vi "test Scaled Parameters for RT to RT.vi"(8 "error in":errorcluster, 11 "Loopback in":refnum<class "Loopback.lvclass">) -> (0 "error out":errorcluster, 3 "Loopback out":refnum<class "Loopback.lvclass">)   [LabVIEW 2020, in "Loopback.lvclass"]
uses:
  Loopback.lvclass
  <vilib>/NI/VeriStand Custom Device Testing Tools/VeriStandTestUtilities/VeriStandTestUtilities.lvlib
  <vilib>/NI VeriStand/Execution/Workspace/NI_VS Workspace ExecutionAPI.lvlib
  <vilib>/NI VeriStand/Execution/Workspace/NI VeriStand - Set Multiple Channel Values.vi
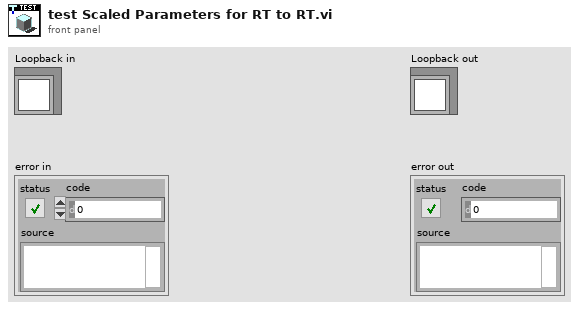
[diagram p1: front panel]
types:
  T1 = typedef "NI_VS Workspace ExecutionAPI.lvlib/WorkspaceAPI.ctl" = refnum<k24>
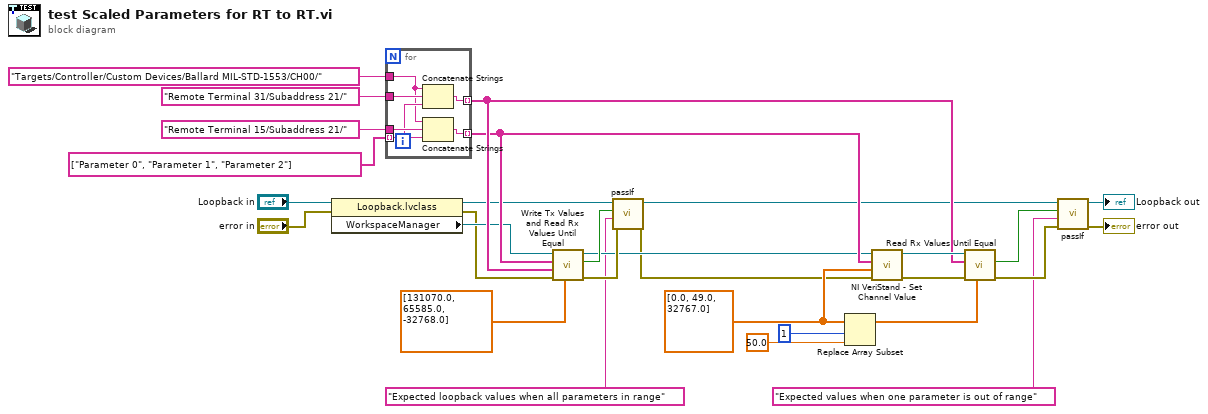
[diagram p0: block diagram]
diagram:
  w27 = dbl[] [0.0, 49.0, 32767.0] ("appended array")
  n1 = property class="Loopback.lvclass"(reference="Loopback in", error in="error in") -> (reference out=w3:refnum<class "Loopback.lvclass">, error out=w4:errorcluster, "WorkspaceManager"=w5:T1)
  n2 = for {
    tunnel: "Remote Terminal 15/Subaddress 21/" ("Channel") -> [w34]
    tunnel: string[] ["Parameter 0", "Parameter 1", "Parameter 2"] ("Channels") -> [w33] mode=indexing
    tunnel: [w35] -> w20 mode=indexing
    tunnel: "Remote Terminal 31/Subaddress 21/" ("Channel") -> [w32]
    tunnel: [w31] -> w21 mode=indexing
    tunnel: "Targets/Controller/Custom Devices/Ballard MIL-STD-1553/CH00/" ("base name for channel aliases") -> [w30]
    n3 = Concatenate Strings(w30, w32, w33) -> (w31:string)
    n4 = Concatenate Strings(w30, w34, w33) -> (w35:string)
  }
  n5 = call <vilib>:"Write Tx Values and Read Rx Values Until Equal.vi"("Tx values"=dbl[] [131070.0, 65585.0, -32768.0] ("appended array"), "error in"=w4, "Rx aliases"=w21, "Tx aliases"=w20, "workspace manager in"=w5) -> ("error out"=w18:errorcluster, "values equal"=w19:bool, "workspace manager out"=w17:T1)  [unwired: 4 in]
  n6 = call-dynamic "passIf.vi"("error in (no error)"=w18, "message (\"\")"="Expected loopback values when all parameters in range" ("message (\"\")"), "pass"=w19, "TestCase in"=w3) -> ("error out"=w11:errorcluster, "TestCase out"=w12:refnum<class "Loopback.lvclass">)  [unwired: 6 in]
  n7 = Replace Array Subset(array=w27, new element=50.0 ("x+y"), index=1) -> (w24:dbl[])
  n8 = call-poly <vilib>:"NI VeriStand - Set Channel Value.vi"("error in (no error)"=w11, "Values"=w27, "Channels"=w20, "WorkspaceManager in"=w17) -> ("error out"=w22:errorcluster, "WorkspaceManager out"=w23:T1)  [unwired: 6 in]
  n9 = call <vilib>:"Read Rx Values Until Equal.vi"("expected values"=w24, "error in"=w22, "Rx aliases"=w21, "workspace manager in"=w23) -> ("error out"=w26:errorcluster, "values equal expected"=w25:bool)  [unwired: 5 in, 1 out]
  n10 = call-dynamic "passIf.vi"("error in (no error)"=w26, "message (\"\")"="Expected values when one parameter is out of range" ("message (\"\")"), "pass"=w25, "TestCase in"=w12) -> ("error out"=→"error out":errorcluster, "TestCase out"=→"Loopback out":refnum<class "Loopback.lvclass">)  [unwired: 6 in]
